vi "ExSubRemoveWarnings.vi"(1 "error in (no error)":errorcluster) -> (0 "error out":errorcluster)   [LabVIEW 2010]
panel:
  # "ExSubRemoveWarnings.vi : this routine takes in an error cluster and returns a clean version\nwith warnings removed. Or stop program if real error."
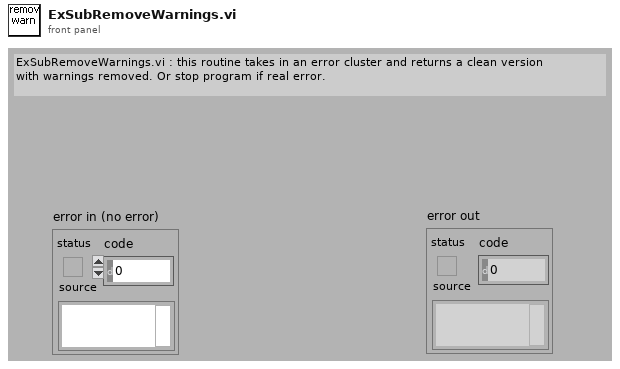
[diagram p1: front panel]
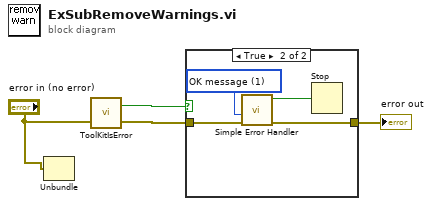
[diagram p0: block diagram]
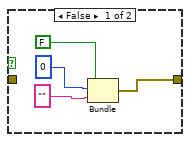
[diagram p2: hidden frame]
diagram:
  n1 = Unbundle("error in (no error)") -> ()  [unwired: 3 out]
  n2 = call <userlib>:"ToolKitIsError.vi"("error in"="error in (no error)") -> ("error out"=w3:errorcluster, "Error Flag"=w4:bool)  [unwired: 1 in]
  n3 = case shown="True" w4 {
    tunnel: w3 -> [_ w12]
    tunnel: [w5 w10] -> w2
    frame False {
      n4 = Bundle(FALSE, 0, "") -> (w5:errorcluster)  [unwired: 1 in]
    }
    frame True {
      w9 = u16 1 items=["no dialog", "OK message", "continue or stop message"] ("type of dialog (OK msg:1)")
      n5 = call <vilib>:"Simple Error Handler.vi"("type of dialog (OK msg:1)"=w9, "error in (no error)"=w12) -> ("error?"=w11:bool, "error out"=w10:errorcluster)  [unwired: 3 in, 3 out]
      n6 = Stop(stop? (T)=w11) -> ()
    }
  }
  "error out" <- w2
